vi "Unsubscribe Client.vi"(8 "error in":errorcluster, 11 "Topic in":refnum<class "Topic.lvclass">) -> (0 "error out":errorcluster, 3 "Topic out":refnum<class "Topic.lvclass">)   [LabVIEW 2014, in "Topic.lvclass"]
uses:
  Topic.lvclass
panel:
  in  "Client":string="Broker"
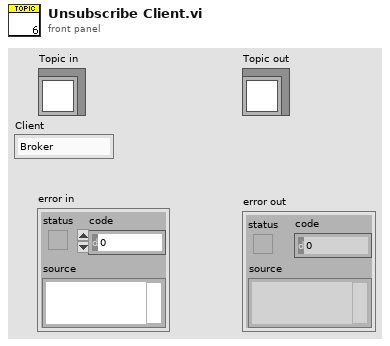
[diagram p1: front panel]
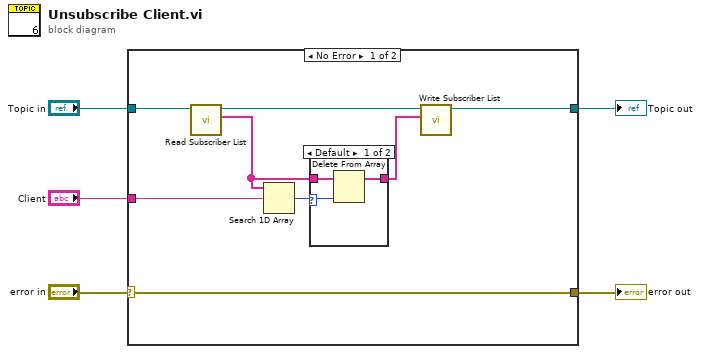
[diagram p0: block diagram]
diagram:
  n1 = case shown="No Error" "error in" {
    selector: "error in" -> [w12 w19]
    tunnel: [w12 w19] -> w4
    tunnel: [w10 w18] -> w2
    tunnel: "Topic in" -> [w13 w18]
    tunnel: "Client" -> [w9 _]
    frame No Error {
      n2 = call-dynamic "Read Subscriber List.vi"("Topic in"=w13) -> ("Subscriber List"=w8:string[], "Topic out"=w11:refnum<class "Topic.lvclass">)  [unwired: 8 in, 1 out]
      n3 = Search 1D Array(1D array=w8, element=w9) -> (index of element=w7:i32)  [unwired: 1 in]
      n4 = case shown="Default" w7 {
        selector: w7 -> [w15 _]
        tunnel: w8 -> [w16 w17]
        tunnel: [w14 w17] -> w6
        frame Default {
          n5 = Delete From Array(array=w16, index=w15) -> (array with subset deleted=w14:string[])  [unwired: 1 in, 1 out]
        }
        frame -1 {
        }
      }
      n6 = call-dynamic "Write Subscriber List.vi"("Subscriber List"=w6, "Topic in"=w11) -> ("Topic out"=w10:refnum<class "Topic.lvclass">)  [unwired: 8 in, 1 out]
    }
    frame Error {
    }
  }
  "error out" <- w4
  "Topic out" <- w2
